vi "Display Errors.vi"(8 "error in (no error)":errorcluster, 10 "Error List":string[](array[string]), 11 "Control Ref":refnum<vi>) -> (0 "error out":errorcluster)   [LabVIEW 2020, in "MacroAssert.lvlib"]
doc: "Populates the string identified by <B>Control Ref</B> with bold-tagged <B>Error List</B>."
uses:
  MacroAssert.lvlib
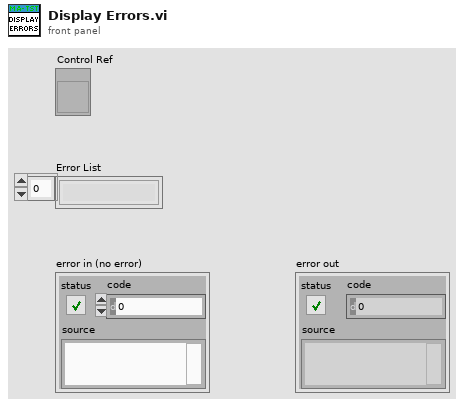
[diagram p1: front panel]
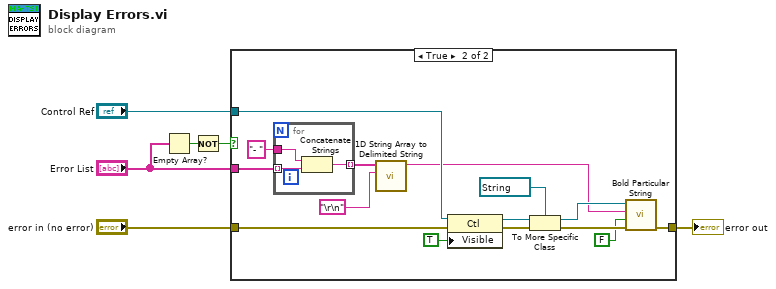
[diagram p0: block diagram]
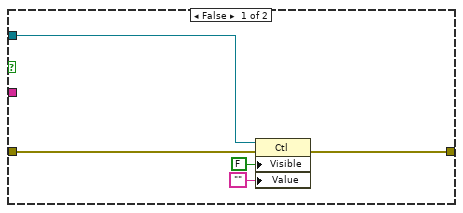
[diagram p2: hidden frame]
diagram:
  n1 = Empty Array?(array="Error List") -> (empty?=w3:bool)
  n2 = Not(x=w3) -> (.not. x?=w1:bool)
  n3 = case shown="True" w1 {
    tunnel: [w8 w26] -> w6
    tunnel: "error in (no error)" -> [w9 w25]
    tunnel: "Control Ref" -> [w7 w24]
    tunnel: "Error List" -> [_ w23]
    frame False {
      n4 = property class="Ctl"(reference=w7, error in=w9, "Visible"=FALSE, "Value"="") -> (error out=w8:errorcluster)  [unwired: 1 out]
    }
    frame True {
      n5 = for {
        tunnel: w23 -> [w29] mode=indexing
        tunnel: [w28] -> w22 mode=indexing
        tunnel: "- " ("string") -> [w27]
        n6 = Concatenate Strings(w27, w29) -> (w28:string)
      }
      n7 = call-poly <vilib>:"1D String Array to Delimited String.vi"("delimiter"="\r\n", "string array"=w22) -> ("delimited string"=w14:string)  [unwired: 9 in]
      n8 = property class="Ctl"(reference=w24, error in=w25, "Visible"=TRUE) -> (reference out=w18:refnum<vi>, error out=w19:errorcluster)
      n9 = To More Specific Class(target class=refnum<vi> refnum ("string refnum"), reference=w18, error in=w19) -> (specific class reference=w15:refnum<vi>, error out=w16:errorcluster)
      n10 = call <vilib>:"Bold Particular String.vi"("error in (no error)"=w16, "resize string? (TRUE)"=FALSE, "text to display"=w14, "string refnum"=w15) -> ("error out"=w26:errorcluster)  [unwired: 6 in, 1 out]
    }
  }
  "error out" <- w6
